vi "gaussian correlation time_flow.vi"() -> ()   [LabVIEW 2016]
panel:
  in  "Correlation Time (s)":dbl
  in  "Max Power (uW/mm^2)":dbl
  in  "Min Power (uW/mm^2)":dbl
  in  "Sigma (uW/mm^2)":dbl
  in  "Offset Power (uW/mm^2)":dbl
  in  "Frames":i32
  in  "Transfer and Run Date Folder After Experiment":bool
  in  "SSH user name":string
  in  "SSH password":string
  in  "Wait before recording (s)":dbl
  in  "Tags":string
  in  "Start Recording":bool
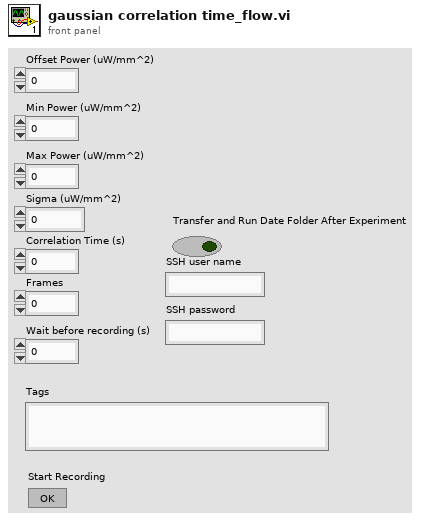
[diagram p1: front panel]
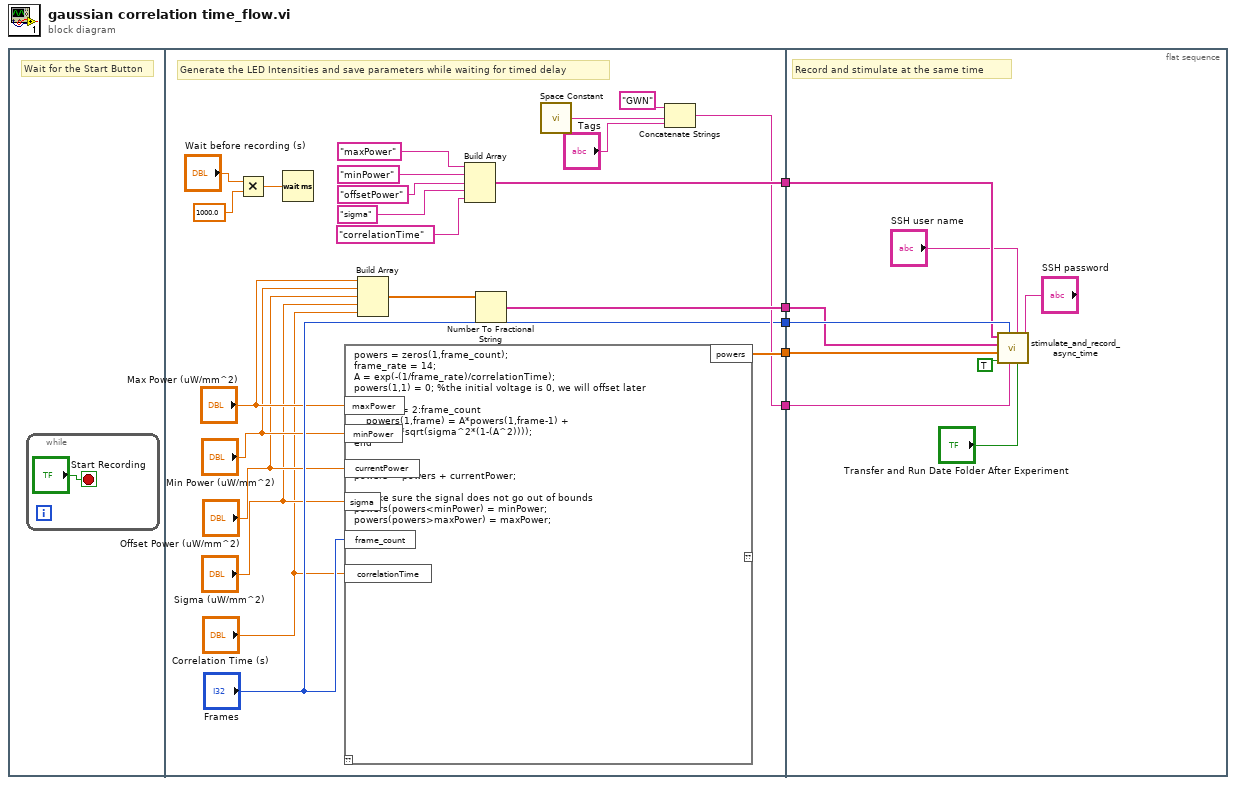
[diagram p0: block diagram]
diagram:
  n1 = flat-sequence {
    tunnel: [w15] -> w5
    tunnel: ["Frames"] -> w4
    tunnel: [w14] -> w3
    tunnel: [w20] -> w2
    tunnel: [w19] -> w1
    tunnel: w5 -> [w34]
    tunnel: w4 -> [w37]
    tunnel: w3 -> [w36]
    tunnel: w2 -> [w33]
    tunnel: w1 -> [w32]
    frame #0 {
      # "Wait for the Start Button"
      n2 = while {
        stop <- "Start Recording" stop-if-true
      }
    }
    frame #1 {
      # "Generate the LED Intensities and save parameters while waiting for timed delay"
      n3 = Multiply(x="Wait before recording (s)", y=1000.0) -> (x*y=w17:dbl)
      n4 = Wait (ms)(milliseconds to wait=w17) -> ()  [unwired: 1 out]
      n5 = script code="powers = zeros(1,frame_count);\nframe_rate = 14;\nA = exp(-(1/frame_rate)/correlationTime);\npowers(1,1) = 0; %the initial voltage is 0, we will offset later\n\nfor frame = 2:frame_count\n    powers(1,frame) = A*powers(1,frame-1) + (randn(1)*sqrt(sigma^2*(1-(A^2))));\nend\n\n%offset\npowers = powers + currentPower;\n\n%make sure the signal does not go out of bounds\npowers(powers<minPower) = minPower;\npowers(powers>maxPower) = maxPower;"("currentPower"="Offset Power (uW/mm^2)", "frame_count"="Frames", "sigma"="Sigma (uW/mm^2)", "minPower"="Min Power (uW/mm^2)", "maxPower"="Max Power (uW/mm^2)", "correlationTime"="Correlation Time (s)") -> ("powers"=w15:dbl[])  [unwired: 1 in, 1 out]
      n6 = Build Array("Max Power (uW/mm^2)", "Min Power (uW/mm^2)", "Offset Power (uW/mm^2)", "Sigma (uW/mm^2)", "Correlation Time (s)") -> (w7:dbl[])
      n7 = Build Array("maxPower", "minPower", "offsetPower", "sigma", "correlationTime") -> (w19:string[])
      n8 = Number To Fractional String(number=w7) -> (F-format string=w20:string[])  [unwired: 3 in]
      n9 = call <vilib>:"Space Constant.vi"() -> ("String"=w27:string)
      n10 = Concatenate Strings("GWN", w27, "Tags") -> (w14:string)
    }
    frame #2 {
      # "Record and stimulate at the same time"
      n11 = call "stimulate_and_record_async_time.vi"("SSH password"="SSH password", "Transfer and Run Date Folder After Experiment"="Transfer and Run Date Folder After Experiment", "SSH user name"="SSH user name", "Tags"=w36, "Frames"=w37, "Convert Power to Voltage"=TRUE, "voltages/power"=w34, "parameters"=w33, "parameters headers"=w32) -> ()  [unwired: 3 in]
    }
  }
